vi "sensor cmd sync get.vi"(10 "current_value":cluster{}, 11 "device_handle":u32) -> (1 "function return":i32, 2 "current_value out":cluster{}, 3 "device_handle out":u32)   [LabVIEW 2019, in "apdm.lvlib"]
doc: "APDM_EXPORT int apdm_sensor_cmd_sync_get(apdm_device_handle_t device_handle, uint64_t *current_value);"
uses:
  apdm.lvlib
  Lee Lab/CP FES Walking 2018/Code/Working/LabVIEW/apdm.dll
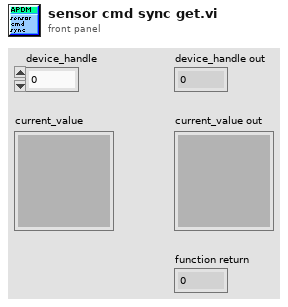
[diagram p1: front panel]
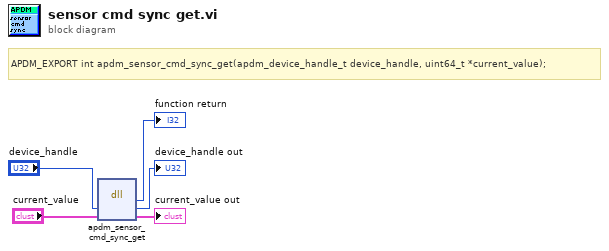
[diagram p0: block diagram]
diagram:
  # "APDM_EXPORT int apdm_sensor_cmd_sync_get(apdm_device_handle_t device_handle, uint64_t *current_value);"
  n1 = dll-call lib="C:/Users/jfalesi/Dropbox/Lee Lab/CP FES Walking 2018/Code/Working/LabVIEW/apdm.*" fn="apdm_sensor_cmd_sync_get"("device_handle"="device_handle", "current_value"="current_value") -> (→"function return":i32, "device_handle"=→"device_handle out":u32, "current_value"=→"current_value out":cluster{})  [unwired: 3 in, 2 out]
